vi "main_CSM.vi"(7 "Name (\"\" to Use UUID)":string="Game") -> ()   [LabVIEW 2025]
doc: "Compact code template used to create a CSM module with a user interface. This template includes a user Event Structure for responding to user actions. The functionality of this template is identical to the CSM User Interface(UI) Module Template VI.\n\n\n> [!NOTE] <b>CSM Naming Rules</b>\n>\n> - CSM module name must be unique. Otherwise, CSM enters a `Critical Error` state.\n> - If the input module name is an empty string (\"\"), the system uses a UUID as the module name. Such a module is marked as standalone mode and does not appear in the module list.\n> - Worker Mode Rule: If the input module name ends with `#`, a worker mode node will be instantiated. Multiple worker mode nodes can form a worker mode module.\n> - Chain of Responsibility Mode Rule: If the input module name ends with `$` followed by a number, a chain of responsibility mode node will be instantiated. Multiple chain of responsibility mode nodes can form a chain of responsibility mode module.\n> - System-Level Module Rule: If the input module name starts with `.`, the module is a system-level module. Under default settings, such modules are not listed by the CSM - List Modules VI and are suitable for instantiating modules that run in the background.\n> - Submodule Rule: `.` is also allowed in a module name to separate the module name into multiple parts. CSM does not have strict rules for submodules. The `.` in the module name only marks the logical relationship between different modules. From an execution perspective, they are considered independent modules. The only difference is that you can obtain a list of logical submodules via the CSM - List Submodules VI.\n\n\n-- <b>Controls</b> --\n- <b>Name (\"\" to use UUID)</b>: CSM module name. Refer to <b>CSM Naming Rules</b> for module naming rules."
uses:
  judgement_note_control.ctl
  <userlib>/_NEVSTOP/Communicable State Machine(CSM)/AdvanceAPI/CSM - Revert Arguments-Safe String.vi
  <userlib>/_NEVSTOP/Communicable State Machine(CSM)/_Shared/Trim Single-line Text.vi
  <userlib>/_NEVSTOP/Communicable State Machine(CSM)/AdvanceAPI/CSM - Break Down Multiple States String.vi
  <userlib>/_NEVSTOP/Communicable State Machine(CSM)/AdvanceAPI/CSM - Compact Multiple States.vi
  <userlib>/_NEVSTOP/Communicable State Machine(CSM)/AdvanceAPI/CSM - Make String Arguments Safe.vi
  <userlib>/_NEVSTOP/Communicable State Machine(CSM)/AdvanceAPI/CSM - Keywords.vi
  <userlib>/_NEVSTOP/Communicable State Machine(CSM)/Communicable State Machine.lvlib
panel:
  in  "StopBeat":bool
  out "BeatActive":bool
  out "BeatInterval Indicator":dbl
  out "T0 indicator":dbl
  out "Play Status":string
  out "array":i32[](array[numeric])
  out "element":i32
  out "Numeric":dbl
  in  "Array":i32[](array[numeric])
  out "Result":string
  out "Current Level 2":string="1" caption="Level"
  in  "Pause":bool
  in  "String":string
  out "Debug Size Equal":bool
  out "Debug Equal":bool
  out "Debug PlayerInput":dbl[](array[numeric])
  out "Debug Notes":dbl[](array[numeric])
  out "Boolean 1":T1
  out "Boolean 4":T1
  out "Boolean 3":T1
  out "Boolean 2":T1
  out "State History":string
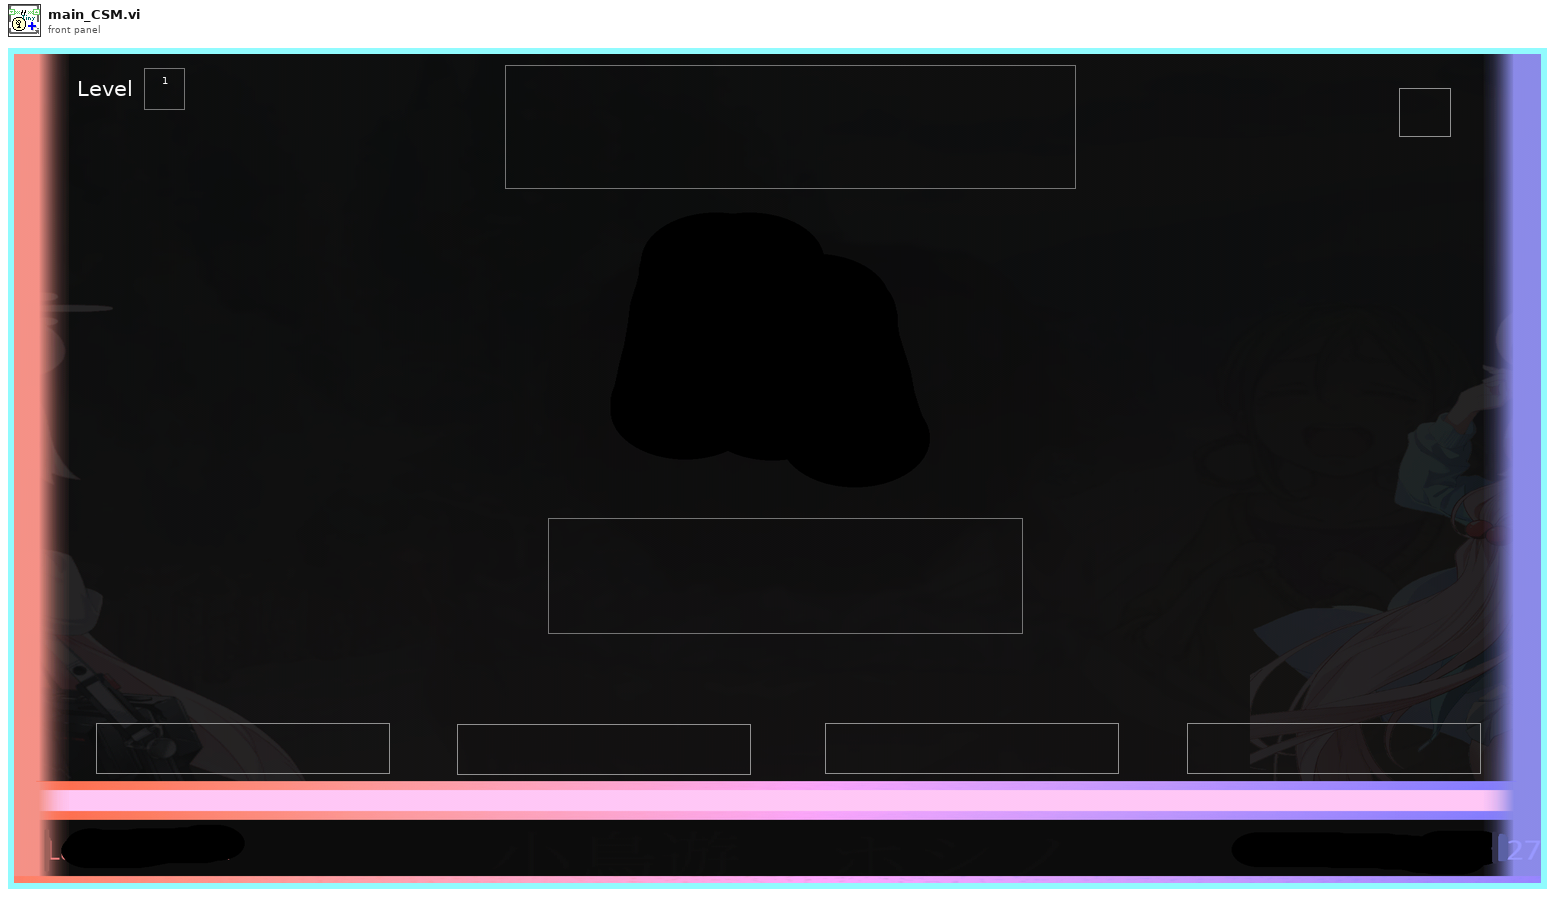
[diagram p1: front panel]
types:
  T1 = typedef "judgement_note_control.ctl" = bool
  T2 = enum32{"Invalid", "Standard", "Closed", "Hidden", "Minimized", "Maximized"}
  T3 = enum32{"invalid app kind", "Development System", "Run Time System", "Student Edition", "Embedded LabVIEW", "Evaluation", "Custom"}
  T4 = typedef "Communicable State Machine.lvlib/_CSM_Response Source Message.ctl" = cluster{"‘State":string, "’Arguments":string, "’Error":errorcluster}
  T5 = cluster{"Core":cluster{"Current VI Reference":refnum<vi>, "Close Panel on Exit?":bool}, "Notes":i32[], "PlayerInput":i32[], "Level":i32, "BeatInterval":i32, "T0":i32, "CurrentTimeout":i32}
  T6 = cluster{"Current VI Reference":refnum<vi>, "Close Panel on Exit?":bool}
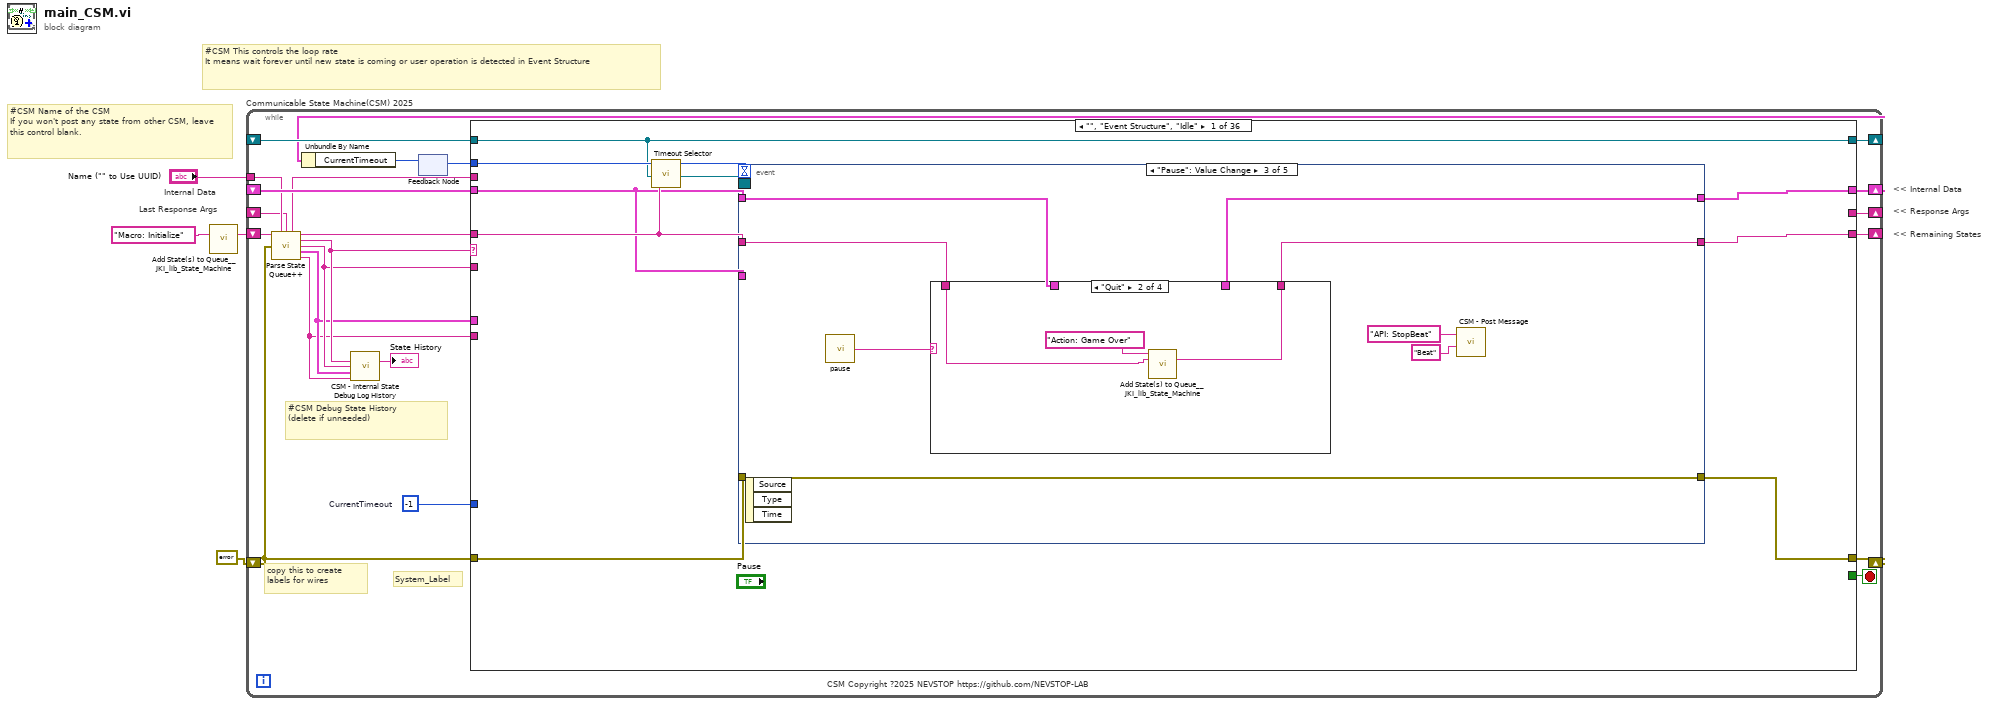
[diagram p0: block diagram]
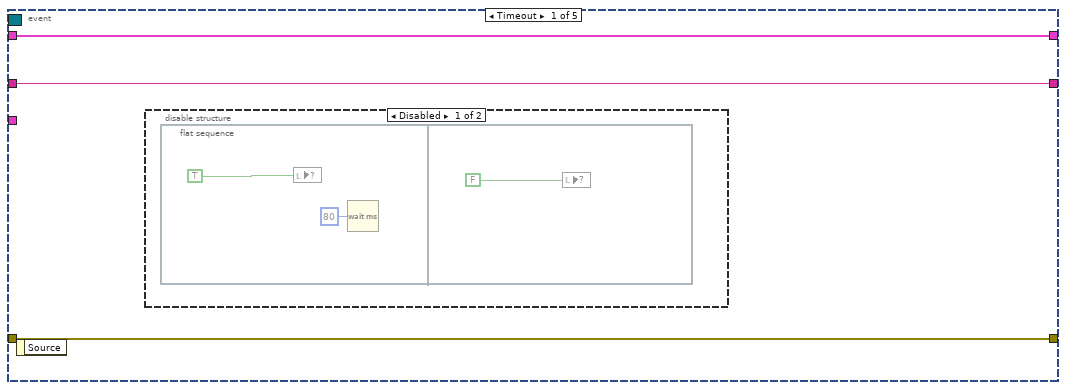
[diagram p2: hidden frame]
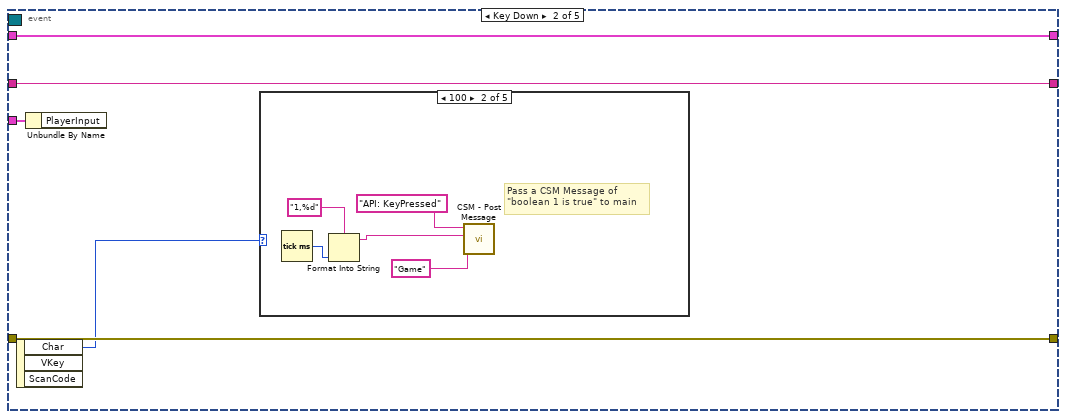
[diagram p4: hidden frame]
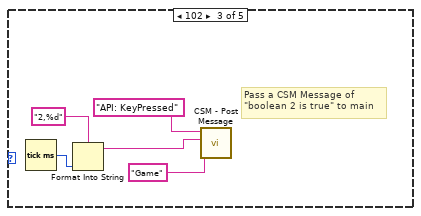
[diagram p6: hidden frame]
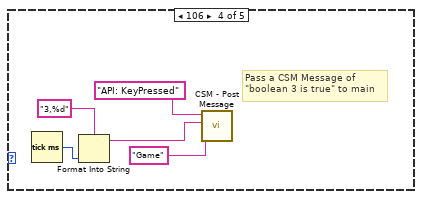
[diagram p7: hidden frame]
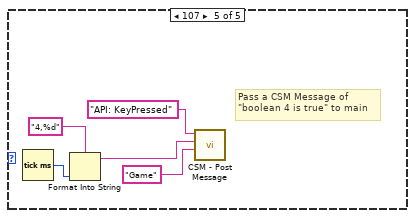
[diagram p8: hidden frame]
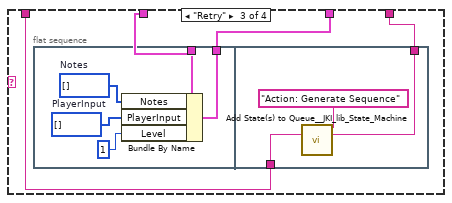
[diagram p10: hidden frame]
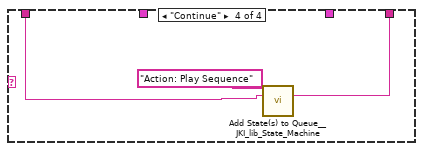
[diagram p11: hidden frame]
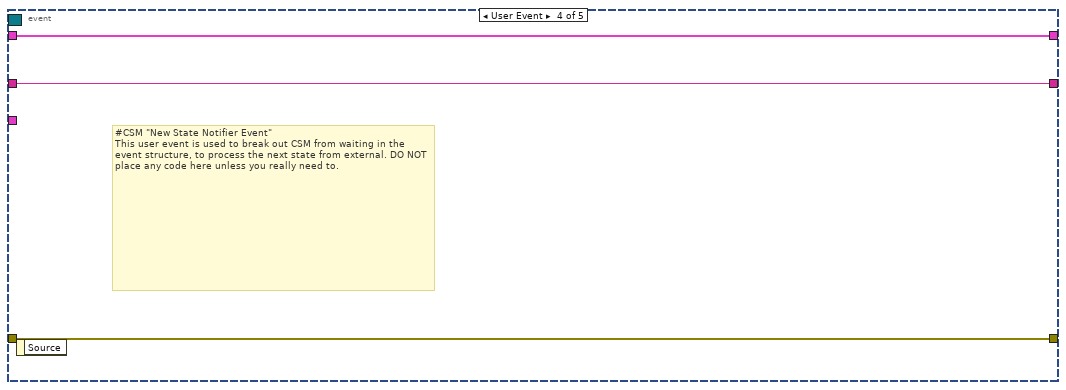
[diagram p12: hidden frame]
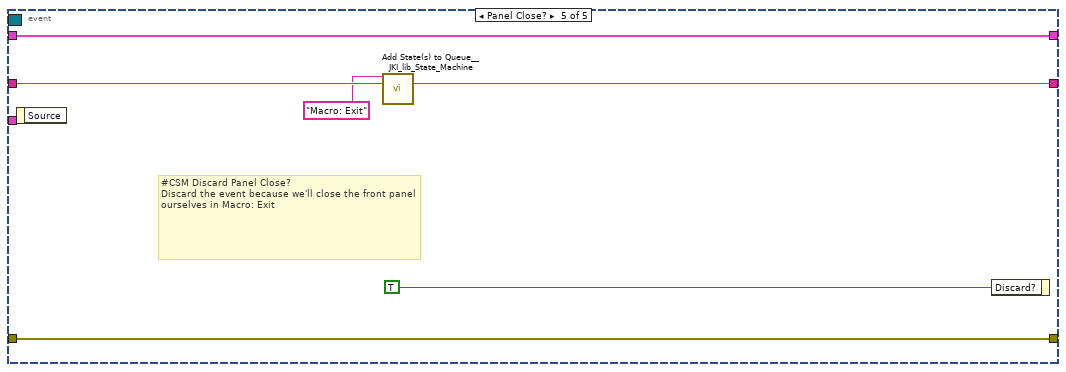
[diagram p13: hidden frame]
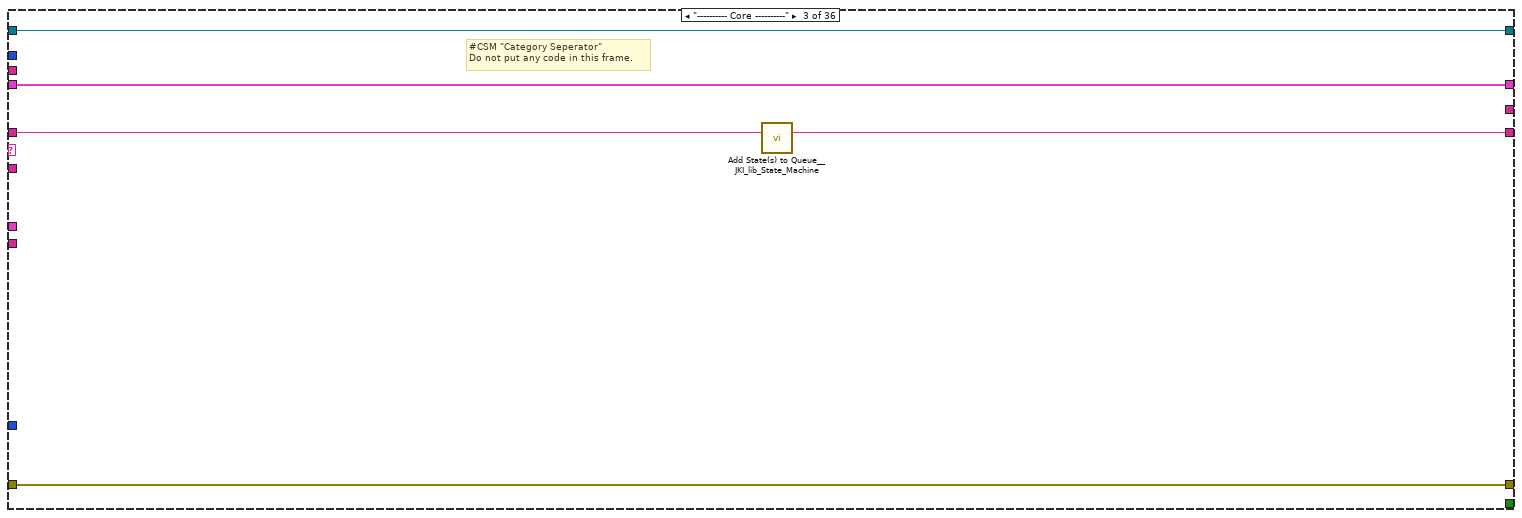
[diagram p15: hidden frame]
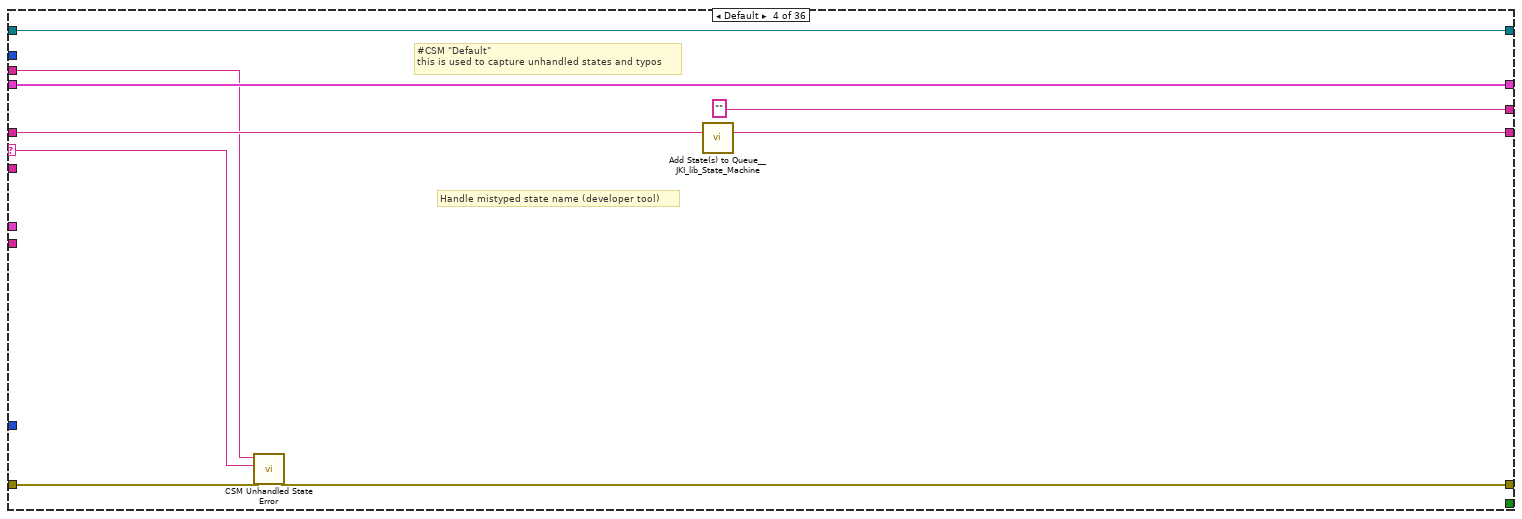
[diagram p16: hidden frame]
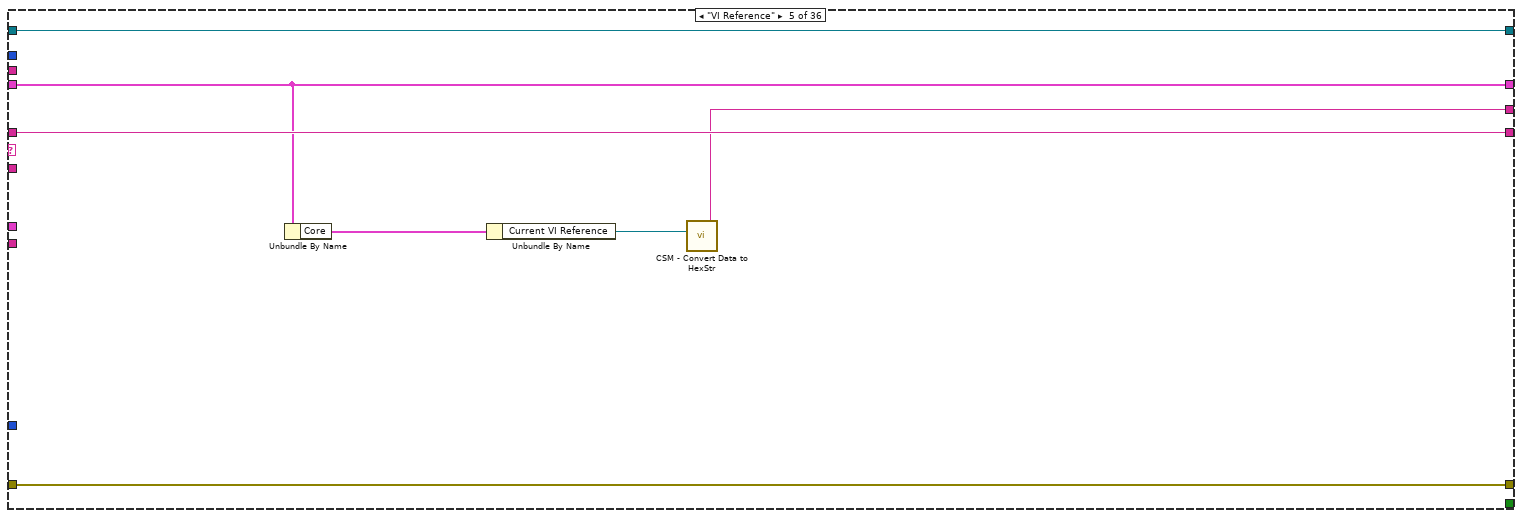
[diagram p17: hidden frame]
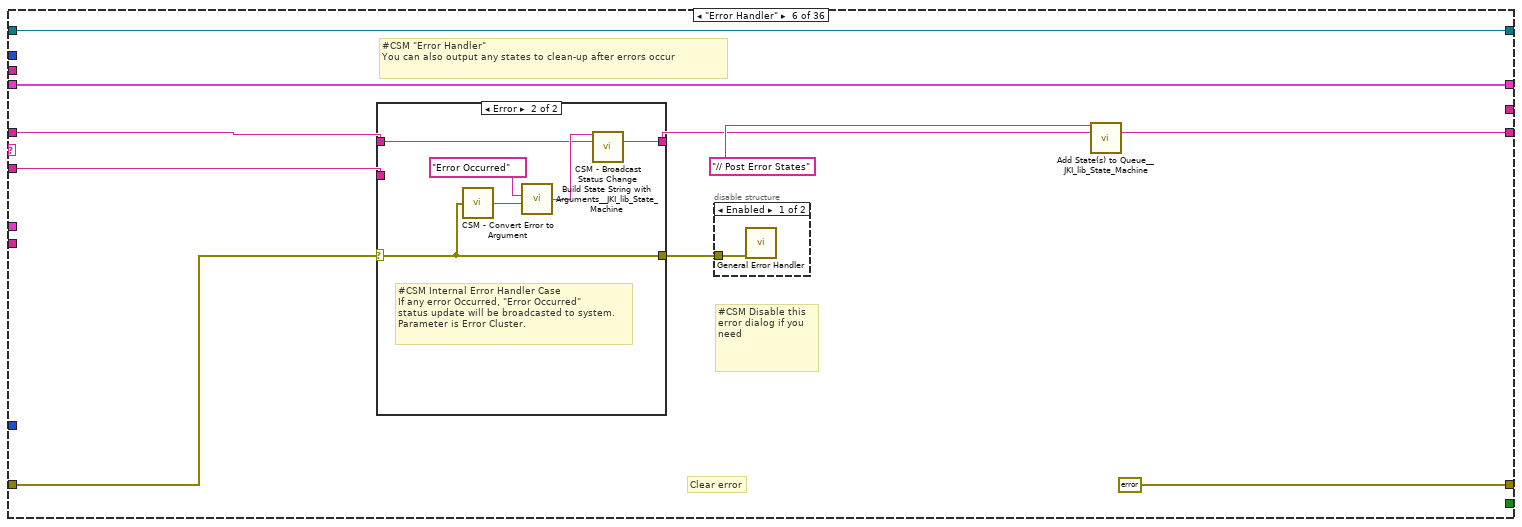
[diagram p18: hidden frame]
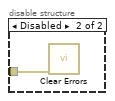
[diagram p19: hidden frame]
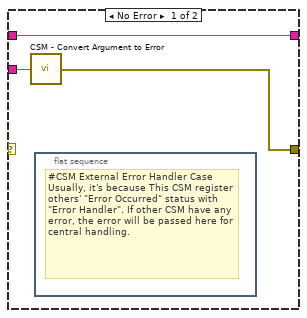
[diagram p20: hidden frame]
diagram:
  # "Last Response Args"
  # "Internal Data"
  # "#CSM Name of the CSM\nIf you won't post any state from other CSM, leave this control blank."
  # "#CSM This controls the loop rate\nIt means wait forever until new state is coming or user operation is detected in Event Structure"
  # "<< Internal Data"
  # "<< Response Args"
  # "<< Remaining States"
  n1 = call <vilib>:"Add State(s) to Queue__JKI_lib_State_Machine.vi"("State(s) in (\"\")"="Macro: Initialize" ("Init State(\"Macro: Initialize\")")) -> ("States Out"=w4:string)  [unwired: 14 in]
  n2 = while "Communicable State Machine(CSM) 2025" {
    shift-right: [w8] -> _
    shift-left: _ -> [w22]
    shift-right: [w24] -> _
    shift-left: errorcluster {"status"=FALSE, "code"=0, "source"=""} ("error out") -> [w21]
    shift-right: [w23] -> _
    shift-left: w4 -> [w25]
    tunnel: "Name (\"\" to Use UUID)" -> [w17]
    shift-right: [w20] -> _
    shift-left: _ -> [w11]
    shift-right: [w19] -> _
    shift-left: _ -> [w18]
    stop <- w5 stop-if-true
    w9 = -1  # CurrentTimeout
    # "#CSM Debug State History\n(delete if unneeded)"
    # "copy this to create labels for wires"
    # "System_Label"
    # "CSM Copyright ?2025 NEVSTOP https://github.com/NEVSTOP-LAB"
    n3 = call <userlib>:"Parse State Queue++.vi"("State Queue"=w25, "Name (\"\" to Use UUID)"=w17, "Response Arguments"=w11, "Previous Error"=w21) -> ("Name Used"=w12:string, "Remaining States"=w26:string, "Current State"=w16:string, "Arguments"=w15:string, "Additional Information"=w14:T4, "Source CSM"=w13:string)  [unwired: 6 in]
    n4 = call <userlib>:"CSM - Internal State Debug Log History.vi"("State"=w16, "Arguments (\"\")"=w15, ">> Response Source Message >>"=w14, "Source (\"\")"=w13) -> ("Debug Log"=→"State History":string)  [unwired: 11 in]
    n5 = feedback #1() -> (w6:i32)  [unwired: 1 in]
    n6 = case shown="\"\", \"Event Structure\", \"Idle\"" w16 {
      selector: w16 -> [_ _ _ w115 _ _ _ _ _ _ _ _ _ _ _ _ _ _ _ _ _ _ _ _ _ _ _ _ _ _ _ _ _ _ _ _]
      tunnel: w26 -> [w28 w106 w112 w120 w127 w133 w156 w162 w169 w178 w191 w206 w212 w217 w229 w236 w241 w248 w252 w258 w264 w271 w287 w357 w363 w375 w378 w394 w420 w427 w442 w447 w457 w470 w551 w604]
      tunnel: w15 -> [_ _ _ _ _ w132 w151 w161 w168 w177 _ _ _ _ _ _ _ _ _ _ _ w266 w281 _ _ _ _ w392 w417 w432 _ _ _ _ _ _]
      tunnel: w22 -> [w27 w105 w109 w118 w126 w137 w157 w164 w171 w180 w190 w199 w210 w214 _ w231 w238 w247 w251 w255 w262 w269 w283 w354 w360 w372 w377 w398 w419 w430 w439 w446 w450 w464 w555 w601]
      tunnel: [w34 w107 w110 w113 w128 errorcluster {"status"=FALSE, "code"=0, "source"=""} ("error out") w152 w159 w166 w183 w192 w203 w209 w215 w227 w232 w239 w242 w250 w256 w261 w267 w284 w355 w361 w373 w379 w402 w421 w435 w440 w448 w455 w468 w563 w611] -> w24
      tunnel: w21 -> [w33 w107 w110 w121 w128 w134 w158 w160 w167 _ w192 w203 w209 w215 w227 w233 w239 _ w253 w256 w261 w268 w285 w355 w361 w373 w379 w402 w421 w435 w440 w448 w455 w468 w563 w611]
      tunnel: [w35 w106 w111 w119 w127 w129 w155 w165 w172 w179 w191 w205 w211 w216 w228 w235 w240 w248 w252 w257 w263 w270 w286 w356 w362 w374 w378 w395 w420 w428 w441 w447 w456 w469 w550 w605] -> w23
      tunnel: [_ _ _ _ _ _ TRUE _ _ _ _ _ TRUE _ _ _ _ _ _ _ _ _ _ _ _ _ _ _ _ _ _ _ _ _ _ _] -> w5
      tunnel: [w32 w105 w109 w118 w126 w137 w157 w164 w171 w181 w190 w204 w210 w214 w219 w231 w238 w247 w251 w255 w262 w269 w283 w354 w360 w372 w377 w396 w419 w429 w439 w446 w449 w465 w556 w607] -> w8
      tunnel: w6 -> [w31 _ _ _ _ _ _ _ _ _ _ _ _ _ _ _ _ _ _ _ _ _ _ _ _ _ _ _ _ _ _ _ _ _ _ _]
      tunnel: w13 -> [_ _ _ _ _ _ _ _ _ w175 _ _ _ _ _ _ _ _ _ _ _ _ _ _ _ _ _ _ _ _ _ _ _ _ _ _]
      tunnel: w14 -> [_ _ _ _ _ _ _ _ _ w182 _ _ _ _ _ _ _ _ _ _ _ _ _ _ _ _ _ _ _ _ _ _ _ _ _ _]
      tunnel: [_ _ _ "" w122 _ _ _ _ _ _ _ _ _ _ _ _ _ _ _ _ _ _ _ _ _ _ "API1 Response" _ w433 _ _ _ _ _ _] -> w20
      tunnel: [w30 w104 w108 w116 w125 w136 w153 w163 w170 w184 w189 w193 w207 w213 w225 w230 w237 w246 w249 w254 w260 w265 w280 w353 w358 w365 w376 w401 w418 w434 w438 w445 w454 w467 w562 w610] -> w19
      tunnel: w18 -> [w30 w104 w108 w116 w125 w136 w153 w163 w170 w184 w189 w193 w207 w213 w225 w230 w237 _ w249 w254 w260 w265 w280 w353 w358 w365 w376 w401 w418 w434 w438 w445 w454 w467 w562 w610]
      tunnel: w12 -> [_ _ _ w114 _ _ w150 _ _ _ _ _ _ _ _ _ _ w245 _ _ _ _ _ _ _ _ _ _ _ _ _ _ _ _ _ _]
      tunnel: w9 -> [_ _ _ _ _ _ _ _ _ _ _ _ _ _ w218 _ _ _ _ _ _ _ _ _ _ _ _ _ _ _ _ _ _ _ _ _]
      frame "", "Event Structure", "Idle" {
        n7 = call <userlib>:"Timeout Selector.vi"("Remaining States"=w28, "Timeout Expected"=w31) -> ("Timeout"=w29:i32)  [unwired: 5 in]
        n8 = event shown="[2] \"Pause\": Value Change" {
          selector: w30 -> [_ _ _ _ _]
          dyn-events: _ -> [_ _ _ _ _]
          timeout: w29 -> [_ _ _ _ _]
          tunnel: w28 -> [w38 w46 w71 w96 w103]
          tunnel: [w38 w46 w70 w96 w102] -> w35
          tunnel: w27 -> [w36 w43 w73 w97 w100]
          tunnel: [w37 w45 w74 w95 w101] -> w34
          tunnel: w33 -> [w37 w45 w74 w95 w101]
          tunnel: [w36 w43 w72 w97 w100] -> w32
          tunnel: w27 -> [_ w44 _ _ _]
          event Timeout {
            n9 = event-data() -> ()  [unwired: 1 in, 1 out]
            n10 = disable-structure shown="Disabled" {
              frame Disabled {
                n11 = flat-sequence {
                  frame #0 {
                    n12 = local write item#-1(TRUE) -> ()
                    n13 = Wait (ms)(milliseconds to wait=u32 80) -> ()  [unwired: 1 out]
                  }
                  frame #1 {
                    n14 = local write item#-1(FALSE) -> ()
                  }
                }
              }
              frame Enabled {
              }
            }
          }
          event Key Down {
            n15 = event-data() -> ("Char"=w42:i16)  [unwired: 1 in, 2 out]
            n16 = Unbundle By Name(w44) -> ()  [unwired: 1 out]
            n17 = case shown="100" w42 {
              frame 0, Default {
              }
              frame 100 {
                # "Pass a CSM Message of \n\"boolean 1 is true\" to main"
                n18 = Tick Count (ms)() -> (millisecond timer value=w49:u32)
                n19 = Format Into String(format string="1,%d", w49) -> (resulting string=w47:string)  [unwired: 2 in, 1 out]
                n20 = call <userlib>:"CSM - Post Message.vi"("Target Module"="Game", "Arguments (\"\")"=w47, "State"="API: KeyPressed") -> ()  [unwired: 8 in, 1 out]
              }
              frame 102 {
                # "Pass a CSM Message of \n\"boolean 2 is true\" to main"
                n21 = Tick Count (ms)() -> (millisecond timer value=w54:u32)
                n22 = Format Into String(format string="2,%d", w54) -> (resulting string=w52:string)  [unwired: 2 in, 1 out]
                n23 = call <userlib>:"CSM - Post Message.vi"("Target Module"="Game", "Arguments (\"\")"=w52, "State"="API: KeyPressed") -> ()  [unwired: 8 in, 1 out]
              }
              frame 106 {
                # "Pass a CSM Message of \n\"boolean 3 is true\" to main"
                n24 = Tick Count (ms)() -> (millisecond timer value=w59:u32)
                n25 = Format Into String(format string="3,%d", w59) -> (resulting string=w57:string)  [unwired: 2 in, 1 out]
                n26 = call <userlib>:"CSM - Post Message.vi"("Target Module"="Game", "Arguments (\"\")"=w57, "State"="API: KeyPressed") -> ()  [unwired: 8 in, 1 out]
              }
              frame 107 {
                # "Pass a CSM Message of \n\"boolean 4 is true\" to main"
                n27 = Tick Count (ms)() -> (millisecond timer value=w64:u32)
                n28 = Format Into String(format string="4,%d", w64) -> (resulting string=w62:string)  [unwired: 2 in, 1 out]
                n29 = call <userlib>:"CSM - Post Message.vi"("Target Module"="Game", "Arguments (\"\")"=w62, "State"="API: KeyPressed") -> ()  [unwired: 8 in, 1 out]
              }
            }
          }
          event "Pause": Value Change {
            n30 = event-data() -> ()  [unwired: 1 in, 3 out]
            n31 = call "pause.vi"() -> ("User's choice"=w69:string)  [unwired: 1 in]
            n32 = case shown="\"Quit\"" w69 {
              tunnel: w73 -> [w76 _ w83 _]
              tunnel: [w76 _ w82 _] -> w72
              tunnel: w71 -> [w75 w78 w81 w93]
              tunnel: [w75 w77 w80 w92] -> w70
              frame "False", Default {
              }
              frame "Quit" {
                n33 = call <vilib>:"Add State(s) to Queue__JKI_lib_State_Machine.vi"("State(s) in Front (\"\")"="Action: Game Over" ("State(s) in Front (\"\")"), "State(s) in (\"\")"=w78) -> ("States Out"=w77:string)  [unwired: 13 in]
              }
              frame "Retry" {
                n34 = flat-sequence {
                  tunnel: w83 -> [w88]
                  tunnel: [w84] -> w82
                  tunnel: w81 -> [w90]
                  tunnel: [w89] -> w80
                  frame #0 {
                    w85 = i32[] []  # PlayerInput
                    w86 = i32[] []  # Notes
                    n35 = Bundle By Name(cluster=w88, "Notes"=w86, "PlayerInput"=w85, "Level"=1) -> (w84:T5)
                  }
                  frame #1 {
                    n36 = call <vilib>:"Add State(s) to Queue__JKI_lib_State_Machine.vi"("State(s) in Front (\"\")"="Action: Generate Sequence" ("State(s) in Front (\"\")"), "State(s) in (\"\")"=w90) -> ("States Out"=w89:string)  [unwired: 13 in]
                  }
                }
              }
              frame "Continue" {
                n37 = call <vilib>:"Add State(s) to Queue__JKI_lib_State_Machine.vi"("State(s) in Front (\"\")"="Action: Play Sequence" ("State(s) in Front (\"\")"), "State(s) in (\"\")"=w93) -> ("States Out"=w92:string)  [unwired: 13 in]
              }
            }
            n38 = call <userlib>:"CSM - Post Message.vi"("Target Module"="Beat", "State"="API: StopBeat") -> ()  [unwired: 9 in, 1 out]
          }
          event User Event {
            # "#CSM \"New State Notifier Event\"\nThis user event is used to break out CSM from waiting in the event structure, to process the next state from external. DO NOT place any code here unless you really need to."
            n39 = event-data() -> ()  [unwired: 1 in, 1 out]
          }
          event Panel Close? {
            # "#CSM Discard Panel Close?\nDiscard the event because we'll close the front panel ourselves in Macro: Exit"
            n40 = event-data() -> ()  [unwired: 1 in, 1 out]
            n41 = call <vilib>:"Add State(s) to Queue__JKI_lib_State_Machine.vi"("State(s) in Front (\"\")"="Macro: Exit", "State(s) in (\"\")"=w103) -> ("States Out"=w102:string)  [unwired: 13 in]
            n42 = event-data("Discard?"=TRUE) -> ()  [unwired: 1 in, 1 out]
          }
        }
      }
      frame "CSM Documentation" {
        # "#CSM README FIRST\n\nCommunicable State Machine(CSM) is a LabVIEW application framework that builds upon JKI State Machine(JKISM). It follows the pattern of JKISM and extends the keywords to describe message communication between modules, including concepts such as Sync-Message, Async-Message, Subscription/Unsubscription of status - essential elements for creating reusable code modules. For more information, please visit the CSM wiki: https://nevstop-lab.github.io/CSM-Wiki/\n\nFor instructions on JKI State Machine, visit: http://jki.net/state-machine/\nFor information about CSM, visit: https://github.com/NEVSTOP-LAB"
        # "#CSM \"Documentation\"\nCase for holding CSM Documenation"
      }
      frame "---------- Core ----------" {
        # "#CSM \"Category Seperator\"\nDo not put any code in this frame."
        n43 = call <vilib>:"Add State(s) to Queue__JKI_lib_State_Machine.vi"("State(s) in (\"\")"=w112) -> ("States Out"=w111:string)  [unwired: 14 in]
      }
      frame Default {
        # "#CSM \"Default\"\nthis is used to capture unhandled states and typos"
        # "Handle mistyped state name (developer tool)"
        n44 = call <userlib>:"CSM Unhandled State Error.vi"("error in (no error)"=w121, "Undefined State"=w115, "CSM Name"=w114) -> ("error out"=w113:errorcluster)  [unwired: 8 in]
        n45 = call <vilib>:"Add State(s) to Queue__JKI_lib_State_Machine.vi"("State(s) in (\"\")"=w120) -> ("States Out"=w119:string)  [unwired: 14 in]
      }
      frame "VI Reference" {
        n46 = Unbundle By Name(w126) -> ("Core"=w124:T6)
        n47 = Unbundle By Name(w124) -> ("Current VI Reference"=w123:refnum<vi>)
        n48 = call <userlib>:"CSM - Convert Data to HexStr.vi"("Variant"=w123) -> ("HEX String (0-9,A-F)"=w122:string)  [unwired: 8 in]
      }
      frame "Error Handler" {
        # "#CSM Disable this error dialog if you need"
        # "#CSM \"Error Handler\"\nYou can also output any states to clean-up after errors occur"
        # "Clear error"
        n49 = case shown="Error" w134 {
          selector: w134 -> [_ w144]
          tunnel: [w143 w146] -> w130
          tunnel: w133 -> [w143 w145]
          tunnel: w132 -> [w142 _]
          tunnel: [w141 w144] -> w135
          frame No Error {
            n50 = call <userlib>:"CSM - Convert Argument to Error.vi"("Argument"=w142) -> ("Error"=w141:errorcluster)  [unwired: 4 in]
            n51 = flat-sequence {
              frame #0 {
                # "#CSM External Error Handler Case\nUsually, it's because This CSM register others' \"Error Occurred\" status with \"Error Handler\". If other CSM have any error, the error will be passed here for central handling."
              }
            }
          }
          frame Error {
            # "#CSM Internal Error Handler Case \nIf any error Occurred, \"Error Occurred\" \nstatus update will be broadcasted to system.\nParameter is Error Cluster."
            n52 = call <userlib>:"CSM - Convert Error to Argument.vi"("Error"=w144) -> ("Argument"=w148:string)  [unwired: 4 in]
            n53 = call <vilib>:"Build State String with Arguments__JKI_lib_State_Machine.vi"("Arguments (\"\")"=w148, "State"="Error Occurred" ("Status with Arguments")) -> ("State with Arguments"=w147:string)  [unwired: 4 in]
            n54 = call <userlib>:"CSM - Broadcast Status Change.vi"("Status With Arguments"=w147, "State Queue"=w145) -> ("Remaining States"=w146:string)  [unwired: 13 in]
          }
        }
        n55 = disable-structure shown="Enabled" {
          disable-tunnel: w135 -> [w139 w140]
          frame Enabled {
            n56 = call <vilib>:"General Error Handler.vi"("error in (no error)"=w139) -> ()  [unwired: 10 in, 5 out]
          }
          frame Disabled {
            n57 = call <vilib>:"Clear Errors.vi"("error in (no error)"=w140) -> ()  [unwired: 5 in, 2 out]
          }
        }
        n58 = call <vilib>:"Add State(s) to Queue__JKI_lib_State_Machine.vi"("State(s) in Front (\"\")"="// Post Error States", "State(s) in (\"\")"=w130) -> ("States Out"=w129:string)  [unwired: 13 in]
      }
      frame "Critical Error" {
        # "#CSM Stop in Critical Error\nWhen Critical Error occurs, Stop the loop immediately. Do NOT change this unless you fully understand the impact."
        # "#CSM \"Critical Error\"\nWhen any un-recoverable error occurs, CSM goes into this case."
        n59 = call <userlib>:"CSM Critical Error.vi"("error in (no error)"=w158, "Arugments (As Reason)"=w151, "CSM Name"=w150) -> ("error out"=w152:errorcluster)  [unwired: 8 in]
        n60 = call <vilib>:"Add State(s) to Queue__JKI_lib_State_Machine.vi"("State(s) in (\"\")"=w156) -> ("States Out"=w155:string)  [unwired: 14 in]
      }
      frame "Target Error" {
        # "#CSM \"Target Error\"\nWhen This CSM try to communicate with an un-existed CSM, This CSM goes into this case."
        n61 = call <userlib>:"CSM Target Error.vi"("error in (no error)"=w160, "Arguments (As CSM Name)"=w161) -> ("error out"=w159:errorcluster)  [unwired: 9 in]
        n62 = call <vilib>:"Add State(s) to Queue__JKI_lib_State_Machine.vi"("State(s) in (\"\")"=w162) -> ("States Out"=w165:string)  [unwired: 14 in]
      }
      frame "Target Timeout Error" {
        # "#CSM \"Target Timeout Error\"\nWhen This CSM could not get the sync-call response in time, This CSM goes into this case."
        n63 = call <userlib>:"CSM Target Timeout Error.vi"("error in (no error)"=w167, "Arguments (As CSM Name)"=w168) -> ("error out"=w166:errorcluster)  [unwired: 9 in]
        n64 = call <vilib>:"Add State(s) to Queue__JKI_lib_State_Machine.vi"("State(s) in (\"\")"=w169) -> ("States Out"=w172:string)  [unwired: 14 in]
      }
      frame "Async Response", "Response" {
        n65 = Unbundle(w182) -> ("‘State"=w176:string, "’Arguments"=w174:string, "’Error"=w173:errorcluster)
        n66 = case shown="Default" w176 {
          tunnel: [w188] -> w183
          tunnel: w173 -> [w188]
          tunnel: [w187] -> w181
          tunnel: w180 -> [w187]
          tunnel: [w185] -> w179
          tunnel: w178 -> [w186]
          tunnel: w177 -> [_]
          tunnel: w175 -> [_]
          tunnel: w174 -> [_]
          frame Default {
            # "#CSM Response Comments\nAfter Message is executed, CSM goes to this state for receive the response.\n    For Async Message(->), \"Async Response\" is used. This CSM will goes to \"Async Message Posted\" immediately and receive the \"Async Response\" after the callee finishes the message.\n    For Sync Message(@),  This CSM will wait until the message is done and immediately goes to \"Response\""
            # "#CSM \"Async Response\"\nHandle Async-call Response (\"Async Response\" for ->)"
            # "#CSM \"Response\"\nHandle Sync-call Response (\"Response\" for -@)"
            n67 = call <vilib>:"Add State(s) to Queue__JKI_lib_State_Machine.vi"("State(s) in (\"\")"=w186) -> ("States Out"=w185:string)  [unwired: 14 in]
          }
        }
      }
      frame "Async Message Posted" {
        # "#CSM \"Async Message Posted\"\nAfter Async Message is posted (-> or ->| ), CSM goes to this state for post-action.\nYou can use Argument - State to tell which Async Message is called."
      }
      frame "Initialize Core Data" {
        # "#CSM \"Initialize Core Data\"\nThis is used to determine panel behavior on exit"
        # "originally closed?"
        # "exe?"
        # "If panel starts closed or is an EXE, then close it when we exit"
        n68 = property class="VI"() -> ("FP.State"=w196:T2)  [unwired: 2 in, 2 out]
        n69 = property class="App"() -> ("App.Kind"=w202:T3)  [unwired: 2 in, 2 out]
        n70 = control-ref of="Current VI Reference"() -> (w197:refnum<vi>)
        n71 = Equal?(x=w196, y=T2."Closed" ("Front Panel Window:State")) -> (x = y?=w194:bool)
        n72 = Equal?(x=w202, y=T3."Run Time System" ("Application:Kind")) -> (x = y?=w200:bool)
        n73 = Or(x=w194, y=w200) -> (x .or. y?=w198:bool)
        n74 = Bundle By Name(cluster=w199, "Core.Current VI Reference"=w197, "Core.Close Panel on Exit?"=w198) -> (w204:T5)
        n75 = call <vilib>:"Add State(s) to Queue__JKI_lib_State_Machine.vi"("State(s) in (\"\")"=w206) -> ("States Out"=w205:string)  [unwired: 14 in]
      }
      frame "Exit" {
        # "#CSM \"Exit\"\nCase for exiting the loop. No errors that occur here will be handled."
        n76 = call <vilib>:"Add State(s) to Queue__JKI_lib_State_Machine.vi"("State(s) in (\"\")"=w212) -> ("States Out"=w211:string)  [unwired: 14 in]
      }
      frame "---------- Data ----------" {
        # "#CSM \"Category Seperator\"\nDo not put any code in this frame."
        n77 = call <vilib>:"Add State(s) to Queue__JKI_lib_State_Machine.vi"("State(s) in (\"\")"=w217) -> ("States Out"=w216:string)  [unwired: 14 in]
      }
      frame "Data: Initialize" {
        w220 = 0  # T0
        w221 = 1  # BeatInterval
        w222 = 1  # Level
        w223 = i32[] []  # PlayerInput
        w224 = i32[] []  # Notes
        w226 = T6 {"Current VI Reference"=refnum, "Close Panel on Exit?"=FALSE}  # Core
        # "#CSM do not delete - used by framework"
        # "#CSM Expand Bundle to add new data elements to shift register data."
        # "#CSM Add new data here."
        # "Initialize the shift-register data, here.\n(data names are defined by what you wire into the bundle function)"
        n78 = Bundle("Core"=w226, "Notes"=w224, "PlayerInput"=w223, "Level"=w222, "BeatInterval"=w221, "T0"=w220, "CurrentTimeout"=w218) -> (w219:T5)  [unwired: 1 in]
        n79 = call <vilib>:"Add State(s) to Queue__JKI_lib_State_Machine.vi"("State(s) in (\"\")"=w229) -> ("States Out"=w228:string)  [unwired: 14 in]
      }
      frame "Data: Cleanup" {
        # "Cleanup any data and references, here.\n(this is called automatically, by the Macro: Exit)"
        n80 = Unbundle By Name(w231) -> ("Core.Current VI Reference"=w234:refnum<vi>)
        n81 = Close Reference(reference=w234, error in (no error)=w233) -> (error out=w232:errorcluster)
        n82 = call <vilib>:"Add State(s) to Queue__JKI_lib_State_Machine.vi"("State(s) in (\"\")"=w236) -> ("States Out"=w235:string)  [unwired: 14 in]
      }
      frame "---------- Events ----------" {
        # "#CSM \"Category Seperator\"\nDo not put any code in this frame."
        n83 = call <vilib>:"Add State(s) to Queue__JKI_lib_State_Machine.vi"("State(s) in (\"\")"=w241) -> ("States Out"=w240:string)  [unwired: 14 in]
      }
      frame "Events: Register" {
        # "#CSM \"Events: Register\"\nRegister user event. New Message Event is registered to break CSM waiting in event structure by default."
        # "#CSM Register New Message Event\nRegister message event to break Waiting in Event structure."
        n84 = call <userlib>:"CSM - Get New State Notifier Event.vi"("Name (\"\" to Use UUID)"=w245) -> ("error out"=w243:errorcluster, "New State Notifier Event"=w244:refnum<user-event>)  [unwired: 9 in]
        n85 = register-events(error in=w243, w244) -> (reference out=w246:refnum<event-registration>, error out=w242:errorcluster)  [unwired: 1 in]
      }
      frame "Events: Unregister" {
        # "#CSM \"Events: Unregister\"\nUnregister user event."
        n86 = Unregister For Events(event registration refnum=w249, error in=w253) -> (error out=w250:errorcluster)
      }
      frame "---------- UI ----------" {
        # "#CSM \"Category Seperator\"\nDo not put any code in this frame."
        n87 = call <vilib>:"Add State(s) to Queue__JKI_lib_State_Machine.vi"("State(s) in (\"\")"=w258) -> ("States Out"=w257:string)  [unwired: 14 in]
      }
      frame "UI: Initialize" {
        # "#CSM \"UI: Initialize\"\nInitialize the User Interface, here.\n(this is called automatically, by the Macro: Init)"
        n88 = property on="String" class="Str"("Key Focus"=TRUE) -> ()  [unwired: 2 in, 2 out]
        n89 = call <vilib>:"Add State(s) to Queue__JKI_lib_State_Machine.vi"("State(s) in (\"\")"=w264) -> ("States Out"=w263:string)  [unwired: 14 in]
      }
      frame "UI: Cursor Set" {
        # "#CSM \"UI: Cursor Set\"\nSet and Unset Cursor Busy.\n(Usage: \"UI: Cursor Set >> Busy|Idle\")"
        # "Argument"
        n90 = disable-structure shown="Default" {
          disable-tunnel: w268 -> [w274 w279]
          disable-tunnel: [w273 w279] -> w267
          disable-tunnel: w266 -> [w272 _]
          frame condition #0 (active) {
            n91 = case shown="\"Idle\", Default" w272 {
              tunnel: w274 -> [w276 w278]
              tunnel: [w275 w277] -> w273
              frame "Idle", Default {
                n92 = call <vilib>:"Unset Busy.vi"("error in (no error)"=w276) -> ("error out"=w275:errorcluster)  [unwired: 10 in]
              }
              frame "Busy" {
                n93 = call <vilib>:"Set Busy.vi"("error in (no error)"=w278) -> ("error out"=w277:errorcluster)  [unwired: 9 in, 1 out]
              }
            }
          }
          frame condition #1 {
          }
        }
        n94 = call <vilib>:"Add State(s) to Queue__JKI_lib_State_Machine.vi"("State(s) in (\"\")"=w271) -> ("States Out"=w270:string)  [unwired: 14 in]
      }
      frame "UI: Front Panel State" {
        # "#CSM \"UI: Front Panel State\"\nSet Front Panel Open or Closed\n(Usage: \"UI: Front Panel State >> Open|Close\")"
        # "Argument"
        n95 = Unbundle By Name(w283) -> ("Core.Current VI Reference"=w282:refnum<vi>)
        n96 = call <vilib>:"Add State(s) to Queue__JKI_lib_State_Machine.vi"("State(s) in (\"\")"=w287) -> ("States Out"=w286:string)  [unwired: 14 in]
        n97 = case shown="\"Open\", \"Standard\", Default" w281 {
          tunnel: w285 -> [w293 w308 w319 w332 w345]
          tunnel: [w295 w309 w321 w334 w347] -> w284
          tunnel: w282 -> [w294 w306 w320 w333 w346]
          frame "Open", "Standard", Default {
            w288 = T2."Maximized" ("State")
            n98 = property class="VI"(reference=w294, error in=w293) -> (reference out=w291:refnum<vi>, error out=w292:errorcluster, "FP.State"=w290:T2)
            n99 = Not Equal?(x=w290, y=w288) -> (x != y?=w289:bool)
            n100 = case shown="True" w289 {
              tunnel: [w299 w301] -> w295
              tunnel: w292 -> [w298 w301]
              tunnel: w291 -> [w297 _]
              tunnel: w288 -> [w296 _]
              frame True {
                n101 = invoke class="VI" method="FP.Open"(reference=w297, error in=w298, "Activate"=TRUE, "State"=w296) -> (error out=w299:errorcluster)  [unwired: 1 in, 4 out]
              }
              frame False {
              }
            }
          }
          frame "Close", "Closed" {
            n102 = property class="VI"(reference=w306, error in=w308) -> (reference out=w305:refnum<vi>, error out=w307:errorcluster, "FP.State"=w303:T2)
            n103 = Not Equal?(x=w303, y=T2."Closed" ("Front Panel Window:State")) -> (x != y?=w302:bool)
            n104 = case shown="False" w302 {
              tunnel: [w310 w313] -> w309
              tunnel: w307 -> [w310 w312]
              tunnel: w305 -> [_ w311]
              frame False {
              }
              frame True {
                n105 = invoke class="VI" method="FP.Close"(reference=w311, error in=w312) -> (error out=w313:errorcluster)  [unwired: 1 in, 2 out]
              }
            }
          }
          frame "Hidden", "Hide" {
            w314 = T2."Hidden" ("State")
            n106 = property class="VI"(reference=w320, error in=w319) -> (reference out=w317:refnum<vi>, error out=w318:errorcluster, "FP.State"=w316:T2)
            n107 = Not Equal?(x=w316, y=w314) -> (x != y?=w315:bool)
            n108 = case shown="True" w315 {
              tunnel: [w325 w326] -> w321
              tunnel: w318 -> [w324 w326]
              tunnel: w317 -> [w323 _]
              tunnel: w314 -> [w322 _]
              frame True {
                n109 = invoke class="VI" method="FP.Open"(reference=w323, error in=w324, "State"=w322) -> (error out=w325:errorcluster)  [unwired: 2 in, 4 out]
              }
              frame False {
              }
            }
          }
          frame "Minimize", "Minimized" {
            w327 = T2."Minimized" ("State")
            n110 = property class="VI"(reference=w333, error in=w332) -> (reference out=w330:refnum<vi>, error out=w331:errorcluster, "FP.State"=w329:T2)
            n111 = Not Equal?(x=w329, y=w327) -> (x != y?=w328:bool)
            n112 = case shown="True" w328 {
              tunnel: [w338 w339] -> w334
              tunnel: w331 -> [w337 w339]
              tunnel: w330 -> [w336 _]
              tunnel: w327 -> [w335 _]
              frame True {
                n113 = invoke class="VI" method="FP.Open"(reference=w336, error in=w337, "State"=w335) -> (error out=w338:errorcluster)  [unwired: 2 in, 4 out]
              }
              frame False {
              }
            }
          }
          frame "Maximize", "Maximized" {
            w340 = T2."Maximized" ("State")
            n114 = property class="VI"(reference=w346, error in=w345) -> (reference out=w343:refnum<vi>, error out=w344:errorcluster, "FP.State"=w342:T2)
            n115 = Not Equal?(x=w342, y=w340) -> (x != y?=w341:bool)
            n116 = case shown="True" w341 {
              tunnel: [w351 w352] -> w347
              tunnel: w344 -> [w350 w352]
              tunnel: w343 -> [w349 _]
              tunnel: w340 -> [w348 _]
              frame True {
                n117 = invoke class="VI" method="FP.Open"(reference=w349, error in=w350, "State"=w348) -> (error out=w351:errorcluster)  [unwired: 2 in, 4 out]
              }
              frame False {
              }
            }
          }
        }
      }
      frame "---------- Macro ----------" {
        # "#CSM \"Category Seperator\"\nDo not put any code in this frame."
        n118 = call <vilib>:"Add State(s) to Queue__JKI_lib_State_Machine.vi"("State(s) in (\"\")"=w357) -> ("States Out"=w356:string)  [unwired: 14 in]
      }
      frame "Macro: Initialize" {
        w359 = "Data: Initialize\nInitialize Core Data\nEvents: Register\nUI: Initialize\nUI: Front Panel State >> Open\nAction: Notify Ready"  # Data: Initialize Initialize Core Data Events: Register UI: Initialize UI: Front Panel State >> Open Action: Notify Ready
        # "#CSM \"Macro: Initialize\"\nInitialization Macro (This is called once, when the VI starts)"
        n119 = call <vilib>:"Add State(s) to Queue__JKI_lib_State_Machine.vi"("State(s) in Front (\"\")"=w359, "State(s) in (\"\")"=w363) -> ("States Out"=w362:string)  [unwired: 13 in]
      }
      frame "Macro: Exit" {
        # "#CSM \"Macro: Exit\"\nExit Macro (This is called once, when the VI exits)"
        n120 = Unbundle By Name(w372) -> ("Core.Close Panel on Exit?"=w371:bool)
        n121 = Select(t="UI: Front Panel State >> Close", s=w371, f="") -> (s? t:f=w368:string)
        n122 = call <vilib>:"Add State(s) to Queue__JKI_lib_State_Machine.vi"("State(s) in Front (\"\")"="//Exit Sub-Modules ", "State(s) in (\"\")"=w368, "State(s) at Back (\"\")"="Data: Cleanup\nEvents: Unregister\nExit") -> ("States Out"=w366:string)  [unwired: 12 in]
        n123 = call <vilib>:"Add State(s) to Queue__JKI_lib_State_Machine.vi"("State(s) in Front (\"\")"=w366, "State(s) in (\"\")"=w375) -> ("States Out"=w374:string)  [unwired: 13 in]
      }
      frame "---------- API ----------" {
        # "#CSM \"Category Seperator\"\nDo not put any code in this frame."
      }
      frame "API: KeyPressed" {
        # "#CSM API Example\nCopy/Rename this case for your own API"
        # "#CSM Response\nConnect this to return the response of your API"
        # "#CSM >> Source CSM >>\nIf you need to tell who triggered this state , use this string. If it's this case itself, this string is \"\"."
        # "#CSM >> Arguments >>\nDeal with the parameter if any"
        n124 = Spreadsheet String To Array(delimiter (Tab)=",", format string="%d", spreadsheet string=w392, array type (2D Dbl)="Array") -> (array=w390:i32[])
        "array" <- w390
        n125 = Index Array(array=w390, index #1=0 ("index"), index #2=1 ("index")) -> (element #1=w387:i32, element #2=w381:i32)
        "Numeric" <- w381
        "element" <- w387
        n126 = Unbundle By Name(w398) -> ("PlayerInput"=w399:i32[])
        n127 = Format Into String(w381) -> (resulting string=w385:string, error out=w386:errorcluster)  [unwired: 3 in]
        n128 = Build Array (concatenate)(w399, w387) -> (w397:i32[])
        n129 = call <userlib>:"CSM - Send Message and Wait for Reply.vi"("Error In (No Error)"=w386, "Target Module"="Judgment", "Arguments (\"\")"=w385, "State"="API: JudgeHit") -> ()  [unwired: 5 in, 3 out]
        n130 = Bundle By Name(cluster=w398, "PlayerInput"=w397) -> (w396:T5)
        n131 = flat-sequence {
          tunnel: w387 -> [w403]
          frame #0 {
            n132 = case shown="4" w403 {
              frame 0, Default {
              }
              frame 1 {
                n133 = local write "Boolean 1"(TRUE) -> ()
                n134 = Wait (ms)(milliseconds to wait=u32 200) -> ()  [unwired: 1 out]
              }
              frame 2 {
                n135 = local write "Boolean 2"(TRUE) -> ()
                n136 = Wait (ms)(milliseconds to wait=u32 200) -> ()  [unwired: 1 out]
              }
              frame 3 {
                n137 = local write "Boolean 3"(TRUE) -> ()
                n138 = Wait (ms)(milliseconds to wait=u32 200) -> ()  [unwired: 1 out]
              }
              frame 4 {
                n139 = local write "Boolean 4"(TRUE) -> ()
                n140 = Wait (ms)(milliseconds to wait=u32 200) -> ()  [unwired: 1 out]
              }
            }
          }
          frame #1 {
            n141 = local write "Boolean 4"(FALSE) -> ()
            n142 = local write "Boolean 3"(FALSE) -> ()
            n143 = local write "Boolean 2"(FALSE) -> ()
            n144 = local write "Boolean 1"(FALSE) -> ()
          }
        }
        n145 = call <vilib>:"Add State(s) to Queue__JKI_lib_State_Machine.vi"("State(s) in Front (\"\")"="Action: Check Input" ("State(s) in Front (\"\")"), "State(s) in (\"\")"=w394) -> ("States Out"=w395:string)  [unwired: 13 in]
      }
      frame "API: HitResult" {
        n146 = case shown="\"Perfect\"" w417 {
          tunnel: [u32 16777225 u32 16731648 u32 16774656 u32 9567230] -> w416
          frame "False", Default {
          }
          frame "Miss" {
          }
          frame "Good" {
          }
          frame "Perfect" {
          }
        }
        n147 = property on="Result" class="Str"("Text.TextColor"=w416) -> ()  [unwired: 2 in, 2 out]
        "Result" <- w417
      }
      frame "API: StartGame" {
        # "#CSM API Example\nCopy/Rename this case for your own API"
        # "unpack Hex String  to Variant\nif complex parameter is needed."
        n148 = Decimal String To Number(string=w432) -> (number=w431:i32)  [unwired: 2 in, 1 out]
        n149 = Bundle By Name(cluster=w430, "BeatInterval"=w431) -> (w429:T5)
        n150 = disable-structure shown="Enabled" {
          disable-tunnel: [w436 "API2 Response"] -> w433
          frame Disabled {
            # "pack variant to hexstr \nif complex response is needed."
            # "complex Response"
            n151 = call <userlib>:"CSM - Convert Data to HexStr.vi"() -> ("HEX String (0-9,A-F)"=w436:string)  [unwired: 9 in]
          }
          frame Enabled {
          }
        }
        n152 = call <vilib>:"Add State(s) to Queue__JKI_lib_State_Machine.vi"("State(s) in Front (\"\")"="Action: Generate Sequence" ("State(s) in Front (\"\")"), "State(s) in (\"\")"=w427) -> ("States Out"=w428:string)  [unwired: 13 in]
      }
      frame "---------- Action ----------" {
        # "#CSM \"Category Seperator\"\nDo not put any code in this frame."
        n153 = call <vilib>:"Add State(s) to Queue__JKI_lib_State_Machine.vi"("State(s) in (\"\")"=w442) -> ("States Out"=w441:string)  [unwired: 14 in]
      }
      frame "Action: Notify Ready" {
        n154 = call <userlib>:"CSM - Post Message.vi"("Target Module"="Menu", "State"="API: GameReady") -> ()  [unwired: 9 in, 1 out]
      }
      frame "Action: Generate Sequence" {
        # "#CSM \"Internal State\"\nThis category is used for holding internal states"
        n155 = Unbundle By Name(w450) -> ("Level"=w452:i32)
        n156 = for {
          N: w452 -> [_]
          tunnel: [w460] -> w451 mode=indexing
          n157 = Random Number (0-1)() -> (number: 0 to 1=w462:dbl)
          n158 = Multiply(x=w462, y=4.0) -> (x*y=w459:dbl)
          n159 = Round Toward +Infinity(x=w459) -> (ceil(x): smallest int >= x=w458:dbl)
          n160 = To Long Integer(number=w458) -> (32bit integer=w460:i32)
        }
        n161 = call <vilib>:"Add State(s) to Queue__JKI_lib_State_Machine.vi"("State(s) in Front (\"\")"="Action: Play Sequence" ("State(s) in Front (\"\")"), "State(s) in (\"\")"=w457) -> ("States Out"=w456:string)  [unwired: 13 in]
        n162 = Bundle By Name(cluster=w450, "Notes"=w451) -> (w449:T5)
      }
      frame "Action: Play Sequence" {
        # "#CSM \"Internal State\"\nThis category is used for holding internal states"
        n163 = flat-sequence {
          tunnel: w464 -> [w475]
          tunnel: [w474] -> w463
          tunnel: w466 -> [w481]
          tunnel: w463 -> [w480]
          tunnel: w463 -> [w479]
          tunnel: w463 -> [w532]
          tunnel: w463 -> [w531]
          tunnel: [w528] -> w465
          frame #0 {
            n164 = Bundle By Name(cluster=w475, "CurrentTimeout"=-1) -> (w474:T5)
            n165 = local write "Play Status"("WATCH") -> ()
            n166 = local write "BeatActive"(FALSE) -> ()
            n167 = Wait (ms)(milliseconds to wait=u32 1000) -> ()  [unwired: 1 out]
            n168 = call <userlib>:"CSM - Post Message.vi"("Target Module"="Beat", "State"="API: StopBeat") -> ()  [unwired: 9 in, 1 out]
          }
          frame #1 {
            n169 = flat-sequence {
              tunnel: w481 -> [w484]
              tunnel: w480 -> [w483]
              tunnel: w479 -> [w482]
              frame #0 {
                n170 = for {
                  tunnel: w484 -> [w487] mode=indexing
                  tunnel: w483 -> [w486]
                  tunnel: w482 -> [w485]
                  n171 = flat-sequence {
                    tunnel: w487 -> [w489]
                    tunnel: w486 -> [w488]
                    tunnel: w485 -> [w521]
                    frame #0 {
                      n172 = case shown="1, Default" w489 {
                        tunnel: w488 -> [w490 w497 w504 w516]
                        frame 1, Default {
                          n173 = Unbundle By Name(w490) -> ("BeatInterval"=w495:i32)
                          n174 = local write "Boolean 1"(TRUE) -> ()
                          n175 = Divide(x=w495, y=3) -> (x/y=w493:dbl)
                          n176 = Multiply(x=w493, y=2.0) -> (x*y=w491:dbl)
                          n177 = Wait (ms)(milliseconds to wait=w491) -> ()  [unwired: 1 out]
                        }
                        frame 2 {
                          n178 = Unbundle By Name(w497) -> ("BeatInterval"=w502:i32)
                          n179 = local write "Boolean 2"(TRUE) -> ()
                          n180 = Divide(x=w502, y=3) -> (x/y=w500:dbl)
                          n181 = Multiply(x=w500, y=2.0) -> (x*y=w498:dbl)
                          n182 = Wait (ms)(milliseconds to wait=w498) -> ()  [unwired: 1 out]
                        }
                        frame 3 {
                          n183 = Unbundle By Name(w504) -> ("BeatInterval"=w509:i32)
                          n184 = local write "Boolean 3"(TRUE) -> ()
                          n185 = Divide(x=w509, y=3) -> (x/y=w507:dbl)
                          n186 = Multiply(x=w507, y=2.0) -> (x*y=w505:dbl)
                          n187 = Wait (ms)(milliseconds to wait=w505) -> ()  [unwired: 1 out]
                        }
                        frame 4 {
                          n188 = Unbundle By Name(w516) -> ("BeatInterval"=w515:i32)
                          n189 = local write "Boolean 4"(TRUE) -> ()
                          n190 = Divide(x=w515, y=3) -> (x/y=w513:dbl)
                          n191 = Multiply(x=w513, y=2.0) -> (x*y=w511:dbl)
                          n192 = Wait (ms)(milliseconds to wait=w511) -> ()  [unwired: 1 out]
                        }
                      }
                    }
                    frame #1 {
                      n193 = local write "Boolean 1"(FALSE) -> ()
                      n194 = local write "Boolean 2"(FALSE) -> ()
                      n195 = local write "Boolean 3"(FALSE) -> ()
                      n196 = local write "Boolean 4"(FALSE) -> ()
                      n197 = Unbundle By Name(w521) -> ("BeatInterval"=w520:i32)
                      n198 = Divide(x=w520, y=3) -> (x/y=w518:dbl)
                      n199 = Wait (ms)(milliseconds to wait=w518) -> ()  [unwired: 1 out]
                    }
                  }
                }
              }
              frame #1 {
                n200 = Wait (ms)(milliseconds to wait=u32 1000) -> ()  [unwired: 1 out]
                n201 = local write "Play Status"("GET READY") -> ()
              }
            }
          }
          frame #2 {
            n202 = flat-sequence {
              tunnel: w532 -> [w543]
              tunnel: w531 -> [w539]
              tunnel: [w539] -> w530
              tunnel: [w538] -> w529
              tunnel: w530 -> [w547]
              tunnel: w529 -> [w546]
              tunnel: [w545] -> w528
              frame #0 {
                # "Pass T0 and BeatInterval\nto Judgment and Beat modules"
                # "T0 + \"BeatInterval\"ms\n per each blinking time"
                n203 = Unbundle By Name(w539) -> ("BeatInterval"=w536:i32)
                "BeatInterval Indicator" <- w536
                n204 = Tick Count (ms)() -> (millisecond timer value=w537:u32)
                "T0 indicator" <- w537
                n205 = Format Into String(format string="%d,%d", w537, w536) -> (resulting string=w533:string)  [unwired: 2 in, 1 out]
                n206 = Bundle By Name(cluster=w543, "T0"=w537) -> (w538:T5)
                n207 = call <userlib>:"CSM - Post Message.vi"("Target Module"="Judgment", "Arguments (\"\")"=w533, "State"="API: BeginInput") -> ()  [unwired: 8 in, 1 out]
                n208 = call <userlib>:"CSM - Post Message.vi"("Target Module"="Beat", "Arguments (\"\")"=w533, "State"="API: StartBeat") -> ()  [unwired: 8 in, 1 out]
              }
              frame #1 {
                n209 = Unbundle By Name(w547) -> ("BeatInterval"=w548:i32)
                n210 = Bundle By Name(cluster=w546, "CurrentTimeout"=w548) -> (w545:T5)
                n211 = local write "Play Status"("YOUR TURN") -> ()
                "BeatActive" <- TRUE
              }
            }
          }
        }
        n212 = Unbundle By Name(w463) -> ("Notes"=w466:i32[])
        n213 = call <vilib>:"Add State(s) to Queue__JKI_lib_State_Machine.vi"("State(s) in (\"\")"=w470) -> ("States Out"=w469:string)  [unwired: 14 in]
      }
      frame "Action: Check Input" {
        # "Check the same index for Notes array"
        # "Array size - 1 to get\nthe last pressed value"
        n214 = Unbundle By Name(w555) -> ("PlayerInput"=w553:i32[])
        n215 = local write "Debug PlayerInput"(w553) -> ()
        n216 = Unbundle By Name(w555) -> ("Notes"=w554:i32[])
        n217 = local write "Debug Notes"(w554) -> ()
        n218 = Array Size(array=w553) -> (size(s)=w557:i32)
        n219 = Subtract(x=w557, y=1) -> (x-y=w558:i32)
        n220 = Index Array(array=w554, index=w558) -> (element=w560:i32)
        n221 = Index Array(array=w553, index=w558) -> (element=w559:i32)
        n222 = Equal?(x=w560, y=w559) -> (x = y?=w552:bool)
        n223 = local write "Debug Equal"(w552) -> ()
        n224 = case shown="False" w552 {
          tunnel: w554 -> [_ w578]
          tunnel: w557 -> [_ w576]
          tunnel: w555 -> [w568 w575]
          tunnel: [w568 w574] -> w556
          tunnel: w555 -> [_ w573]
          tunnel: w551 -> [w566 w571]
          tunnel: [w567 w570] -> w550
          frame False {
            n225 = call <vilib>:"Add State(s) to Queue__JKI_lib_State_Machine.vi"("State(s) in Front (\"\")"="Action: Game Over" ("State(s) in Front (\"\")"), "State(s) in (\"\")"=w566) -> ("States Out"=w567:string)  [unwired: 13 in]
            n226 = call <userlib>:"CSM - Post Message.vi"("Target Module"="Beat", "State"="API: StopBeat") -> ()  [unwired: 9 in, 1 out]
          }
          frame True {
            # "Check if Notes and PlayerInput\nhave the same array size"
            n227 = Array Size(array=w578) -> (size(s)=w577:i32)
            n228 = Equal?(x=w577, y=w576) -> (x = y?=w572:bool)
            n229 = local write "Debug Size Equal"(w572) -> ()
            n230 = case shown="True" w572 {
              tunnel: w575 -> [w580 w593]
              tunnel: [w580 w592] -> w574
              tunnel: w573 -> [_ w589]
              tunnel: w571 -> [w579 w586]
              tunnel: [w579 w585] -> w570
              frame False {
              }
              frame True {
                # "Display the \ncurrent level reached"
                # "Clear notes and player input,\nlevel up, clear timeout"
                n231 = Unbundle By Name(w589) -> ("Level"=w588:i32)
                n232 = Add(x=1, y=w588) -> (x+y=w583:i32)
                n233 = Bundle By Name(cluster=w593, "Notes"=i32[] [], "PlayerInput"=i32[] [], "Level"=w583, "CurrentTimeout"=-1) -> (w592:T5)
                n234 = Format Into String(w583) -> (resulting string=→"Current Level 2":string)  [unwired: 3 in, 1 out]
                n235 = call <vilib>:"Add State(s) to Queue__JKI_lib_State_Machine.vi"("State(s) in Front (\"\")"="Action: Generate Sequence" ("State(s) in (\"\")"), "State(s) in (\"\")"=w586) -> ("States Out"=w585:string)  [unwired: 13 in]
              }
            }
          }
        }
      }
      frame "Action: Game Over" {
        # "Close game page when game over\nand return to menu page"
        # "Clear notes and player inputs,\nlevel restart from 1,\nclear timeout"
        n236 = local write "BeatActive"(FALSE) -> ()
        n237 = Bundle By Name(cluster=w601, "Core.Close Panel on Exit?"=TRUE) -> (w600:T5)
        n238 = call <userlib>:"CSM - Post Message.vi"("Target Module"="Menu", "State"="API: GameReady") -> ()  [unwired: 9 in, 1 out]
        n239 = call <userlib>:"CSM - Post Message.vi"("Target Module"="Beat", "State"="API: StopBeat") -> ()  [unwired: 9 in, 1 out]
        n240 = Bundle By Name(cluster=w600, "Notes"=i32[] [], "PlayerInput"=i32[] [], "Level"=1, "CurrentTimeout"=-1) -> (w607:T5)
        n241 = call <vilib>:"Add State(s) to Queue__JKI_lib_State_Machine.vi"("State(s) in Front (\"\")"="Macro: Exit" ("State(s) in Front (\"\")"), "State(s) in (\"\")"=w604) -> ("States Out"=w605:string)  [unwired: 13 in]
      }
    }
    n242 = Unbundle By Name(w8) -> ("CurrentTimeout"=w7:i32)
    n243 = feedback-in #1(w7) -> ()
  }
